vi "Paths to Commands_new.vi"(2 "Path":T4(array[cluster]), 3 "Path Properties":T1(array[cluster])=[{"Speed (um/s)"=0.4, "Direction"=0, "Orientation (For Filled)"=enum."Vertical", "Curve smooth Segments"=30.0, "Fill in spacing (um)"=0.3, "Start and End voltage"=[{"Numeric"=10.0, "Numeric 2"=10.0}, {"Numeric"=-10.0, "Numeric 2"=-10.0}, {"Numeric"=10.0, "Numeric 2"=10.0}], "Same Voltage"=TRUE, "Function Genrator?"=TRUE}, {"Speed (um/s)"=0.4, "Direction"=0, "Orientation (For Filled)"=enum."Vertical", "Curve smooth Segments"=30.0, "Fill in spacing (um)"=0.3, "Start and End voltage"=[{"Numeric"=10.0, "Numeric 2"=10.0}, {"Numeric"=-10.0, "Numeric 2"=-10.0}, {"Numeric"=10.0, "Numeric 2"=10.0}], "Same Voltage"=TRUE, "Function Genrator?"=TRUE}, {"Speed (um/s)"=0.4, "Direction"=0, "Orientation (For Filled)"=enum."Vertical", "Curve smooth Segments"=30.0, "Fill in spacing (um)"=0.3, "Start and End voltage"=[{"Numeric"=10.0, "Numeric 2"=10.0}, {"Numeric"=-10.0, "Numeric 2"=-10.0}, {"Numeric"=10.0, "Numeric 2"=10.0}], "Same Voltage"=TRUE, "Function Genrator?"=TRUE}, {"Speed (um/s)"=0.4, "Direction"=0, "Orientation (For Filled)"=enum."Vertical", "Curve smooth Segments"=30.0, "Fill in spacing (um)"=0.3, "Start and End voltage"=[{"Numeric"=10.0, "Numeric 2"=10.0}, {"Numeric"=-10.0, "Numeric 2"=-10.0}, {"Numeric"=10.0, "Numeric 2"=10.0}], "Same Voltage"=TRUE, "Function Genrator?"=TRUE}, {"Speed (um/s)"=0.4, "Direction"=0, "Orientation (For Filled)"=enum."Vertical", "Curve smooth Segments"=30.0, "Fill in spacing (um)"=0.3, "Start and End voltage"=[{"Numeric"=10.0, "Numeric 2"=10.0}, {"Numeric"=-10.0, "Numeric 2"=-10.0}, {"Numeric"=10.0, "Numeric 2"=10.0}], "Same Voltage"=TRUE, "Function Genrator?"=TRUE}, {"Speed (um/s)"=0.4, "Direction"=0, "Orientation (For Filled)"=enum."Vertical", "Curve smooth Segments"=30.0, "Fill in spacing (um)"=0.3, "Start and End voltage"=[{"Numeric"=10.0, "Numeric 2"=10.0}, {"Numeric"=-10.0, "Numeric 2"=-10.0}, {"Numeric"=10.0, "Numeric 2"=10.0}], "Same Voltage"=TRUE, "Function Genrator?"=TRUE}, {"Speed (um/s)"=0.4, "Direction"=0, "Orientation (For Filled)"=enum."Vertical", "Curve smooth Segments"=30.0, "Fill in spacing (um)"=0.3, "Start and End voltage"=[{"Numeric"=10.0, "Numeric 2"=10.0}, {"Numeric"=-10.0, "Numeric 2"=-10.0}, {"Numeric"=10.0, "Numeric 2"=10.0}], "Same Voltage"=TRUE, "Function Genrator?"=TRUE}, {"Speed (um/s)"=0.4, "Direction"=0, "Orientation (For Filled)"=enum."Vertical", "Curve smooth Segments"=30.0, "Fill in spacing (um)"=0.3, "Start and End voltage"=[{"Numeric"=10.0, "Numeric 2"=10.0}, {"Numeric"=-10.0, "Numeric 2"=-10.0}, {"Numeric"=10.0, "Numeric 2"=10.0}], "Same Voltage"=TRUE, "Function Genrator?"=TRUE}, {"Speed (um/s)"=0.4, "Direction"=0, "Orientation (For Filled)"=enum."Vertical", "Curve smooth Segments"=30.0, "Fill in spacing (um)"=0.3, "Start and End voltage"=[{"Numeric"=10.0, "Numeric 2"=10.0}, {"Numeric"=-10.0, "Numeric 2"=-10.0}, {"Numeric"=10.0, "Numeric 2"=10.0}], "Same Voltage"=TRUE, "Function Genrator?"=TRUE}, {"Speed (um/s)"=0.4, "Direction"=0, "Orientation (For Filled)"=enum."Vertical", "Curve smooth Segments"=30.0, "Fill in spacing (um)"=0.3, "Start and End voltage"=[{"Numeric"=10.0, "Numeric 2"=10.0}, {"Numeric"=-10.0, "Numeric 2"=-10.0}, {"Numeric"=10.0, "Numeric 2"=10.0}], "Same Voltage"=TRUE, "Function Genrator?"=TRUE}, {"Speed (um/s)"=0.4, "Direction"=0, "Orientation (For Filled)"=enum."Vertical", "Curve smooth Segments"=30.0, "Fill in spacing (um)"=0.3, "Start and End voltage"=[{"Numeric"=10.0, "Numeric 2"=10.0}, {"Numeric"=-10.0, "Numeric 2"=-10.0}, {"Numeric"=10.0, "Numeric 2"=10.0}], "Same Voltage"=TRUE, "Function Genrator?"=TRUE}, {"Speed (um/s)"=0.4, "Direction"=0, "Orientation (For Filled)"=enum."Vertical", "Curve smooth Segments"=30.0, "Fill in spacing (um)"=0.3, "Start and End voltage"=[{"Numeric"=10.0, "Numeric 2"=10.0}, {"Numeric"=-10.0, "Numeric 2"=-10.0}, {"Numeric"=10.0, "Numeric 2"=10.0}], "Same Voltage"=TRUE, "Function Genrator?"=TRUE}, {"Speed (um/s)"=0.4, "Direction"=0, "Orientation (For Filled)"=enum."Vertical", "Curve smooth Segments"=30.0, "Fill in spacing (um)"=0.3, "Start and End voltage"=[{"Numeric"=10.0, "Numeric 2"=10.0}, {"Numeric"=-10.0, "Numeric 2"=-10.0}, {"Numeric"=10.0, "Numeric 2"=10.0}], "Same Voltage"=TRUE, "Function Genrator?"=TRUE}, {"Speed (um/s)"=0.4, "Direction"=0, "Orientation (For Filled)"=enum."Vertical", "Curve smooth Segments"=30.0, "Fill in spacing (um)"=0.3, "Start and End voltage"=[{"Numeric"=10.0, "Numeric 2"=10.0}, {"Numeric"=-10.0, "Numeric 2"=-10.0}, {"Numeric"=10.0, "Numeric 2"=10.0}], "Same Voltage"=TRUE, "Function Genrator?"=TRUE}, {"Speed (um/s)"=0.4, "Direction"=0, "Orientation (For Filled)"=enum."Vertical", "Curve smooth Segments"=30.0, "Fill in spacing (um)"=0.3, "Start and End voltage"=[{"Numeric"=10.0, "Numeric 2"=10.0}, {"Numeric"=-10.0, "Numeric 2"=-10.0}, {"Numeric"=10.0, "Numeric 2"=10.0}], "Same Voltage"=TRUE, "Function Genrator?"=TRUE}, {"Speed (um/s)"=0.4, "Direction"=0, "Orientation (For Filled)"=enum."Vertical", "Curve smooth Segments"=30.0, "Fill in spacing (um)"=0.3, "Start and End voltage"=[{"Numeric"=10.0, "Numeric 2"=10.0}, {"Numeric"=-10.0, "Numeric 2"=-10.0}, {"Numeric"=10.0, "Numeric 2"=10.0}], "Same Voltage"=TRUE, "Function Genrator?"=TRUE}, {"Speed (um/s)"=0.4, "Direction"=0, "Orientation (For Filled)"=enum."Vertical", "Curve smooth Segments"=30.0, "Fill in spacing (um)"=0.3, "Start and End voltage"=[{"Numeric"=10.0, "Numeric 2"=10.0}, {"Numeric"=-10.0, "Numeric 2"=-10.0}, {"Numeric"=10.0, "Numeric 2"=10.0}], "Same Voltage"=TRUE, "Function Genrator?"=TRUE}, {"Speed (um/s)"=0.4, "Direction"=0, "Orientation (For Filled)"=enum."Vertical", "Curve smooth Segments"=30.0, "Fill in spacing (um)"=0.3, "Start and End voltage"=[{"Numeric"=10.0, "Numeric 2"=10.0}, {"Numeric"=-10.0, "Numeric 2"=-10.0}, {"Numeric"=10.0, "Numeric 2"=10.0}], "Same Voltage"=TRUE, "Function Genrator?"=TRUE}, {"Speed (um/s)"=0.4, "Direction"=0, "Orientation (For Filled)"=enum."Vertical", "Curve smooth Segments"=30.0, "Fill in spacing (um)"=0.3, "Start and End voltage"=[{"Numeric"=10.0, "Numeric 2"=10.0}, {"Numeric"=-10.0, "Numeric 2"=-10.0}, {"Numeric"=10.0, "Numeric 2"=10.0}], "Same Voltage"=TRUE, "Function Genrator?"=TRUE}, {"Speed (um/s)"=0.4, "Direction"=0, "Orientation (For Filled)"=enum."Vertical", "Curve smooth Segments"=30.0, "Fill in spacing (um)"=0.3, "Start and End voltage"=[{"Numeric"=10.0, "Numeric 2"=10.0}, {"Numeric"=-10.0, "Numeric 2"=-10.0}, {"Numeric"=10.0, "Numeric 2"=10.0}], "Same Voltage"=TRUE, "Function Genrator?"=TRUE}, {"Speed (um/s)"=0.4, "Direction"=0, "Orientation (For Filled)"=enum."Vertical", "Curve smooth Segments"=30.0, "Fill in spacing (um)"=0.3, "Start and End voltage"=[{"Numeric"=10.0, "Numeric 2"=10.0}, {"Numeric"=-10.0, "Numeric 2"=-10.0}, {"Numeric"=10.0, "Numeric 2"=10.0}], "Same Voltage"=TRUE, "Function Genrator?"=TRUE}, {"Speed (um/s)"=0.4, "Direction"=0, "Orientation (For Filled)"=enum."Vertical", "Curve smooth Segments"=30.0, "Fill in spacing (um)"=0.3, "Start and End voltage"=[{"Numeric"=10.0, "Numeric 2"=10.0}, {"Numeric"=-10.0, "Numeric 2"=-10.0}, {"Numeric"=10.0, "Numeric 2"=10.0}], "Same Voltage"=TRUE, "Function Genrator?"=TRUE}, {"Speed (um/s)"=0.4, "Direction"=0, "Orientation (For Filled)"=enum."Vertical", "Curve smooth Segments"=30.0, "Fill in spacing (um)"=0.3, "Start and End voltage"=[{"Numeric"=10.0, "Numeric 2"=10.0}, {"Numeric"=-10.0, "Numeric 2"=-10.0}, {"Numeric"=10.0, "Numeric 2"=10.0}], "Same Voltage"=TRUE, "Function Genrator?"=TRUE}, {"Speed (um/s)"=0.4, "Direction"=0, "Orientation (For Filled)"=enum."Vertical", "Curve smooth Segments"=30.0, "Fill in spacing (um)"=0.3, "Start and End voltage"=[{"Numeric"=10.0, "Numeric 2"=10.0}, {"Numeric"=-10.0, "Numeric 2"=-10.0}, {"Numeric"=10.0, "Numeric 2"=10.0}], "Same Voltage"=TRUE, "Function Genrator?"=TRUE}, {"Speed (um/s)"=0.4, "Direction"=0, "Orientation (For Filled)"=enum."Vertical", "Curve smooth Segments"=30.0, "Fill in spacing (um)"=0.3, "Start and End voltage"=[{"Numeric"=10.0, "Numeric 2"=10.0}, {"Numeric"=-10.0, "Numeric 2"=-10.0}, {"Numeric"=10.0, "Numeric 2"=10.0}], "Same Voltage"=TRUE, "Function Genrator?"=TRUE}, {"Speed (um/s)"=0.4, "Direction"=0, "Orientation (For Filled)"=enum."Vertical", "Curve smooth Segments"=30.0, "Fill in spacing (um)"=0.3, "Start and End voltage"=[{"Numeric"=10.0, "Numeric 2"=10.0}, {"Numeric"=-10.0, "Numeric 2"=-10.0}, {"Numeric"=10.0, "Numeric 2"=10.0}], "Same Voltage"=TRUE, "Function Genrator?"=TRUE}, {"Speed (um/s)"=0.4, "Direction"=0, "Orientation (For Filled)"=enum."Vertical", "Curve smooth Segments"=30.0, "Fill in spacing (um)"=0.3, "Start and End voltage"=[{"Numeric"=10.0, "Numeric 2"=10.0}, {"Numeric"=-10.0, "Numeric 2"=-10.0}, {"Numeric"=10.0, "Numeric 2"=10.0}], "Same Voltage"=TRUE, "Function Genrator?"=TRUE}, {"Speed (um/s)"=0.4, "Direction"=0, "Orientation (For Filled)"=enum."Vertical", "Curve smooth Segments"=30.0, "Fill in spacing (um)"=0.3, "Start and End voltage"=[{"Numeric"=10.0, "Numeric 2"=10.0}, {"Numeric"=-10.0, "Numeric 2"=-10.0}, {"Numeric"=10.0, "Numeric 2"=10.0}], "Same Voltage"=TRUE, "Function Genrator?"=TRUE}, {"Speed (um/s)"=0.4, "Direction"=0, "Orientation (For Filled)"=enum."Vertical", "Curve smooth Segments"=30.0, "Fill in spacing (um)"=0.3, "Start and End voltage"=[{"Numeric"=10.0, "Numeric 2"=10.0}, {"Numeric"=-10.0, "Numeric 2"=-10.0}, {"Numeric"=10.0, "Numeric 2"=10.0}], "Same Voltage"=TRUE, "Function Genrator?"=TRUE}, {"Speed (um/s)"=0.4, "Direction"=0, "Orientation (For Filled)"=enum."Vertical", "Curve smooth Segments"=30.0, "Fill in spacing (um)"=0.3, "Start and End voltage"=[{"Numeric"=10.0, "Numeric 2"=10.0}, {"Numeric"=-10.0, "Numeric 2"=-10.0}, {"Numeric"=10.0, "Numeric 2"=10.0}], "Same Voltage"=TRUE, "Function Genrator?"=TRUE}] {"Direction" items=["Forward", "Backward"]}, 4 "error in (no error)":errorcluster) -> (0 "Lithography information":T2(array[cluster]), 1 "error out":errorcluster)   [LabVIEW 2013]
doc: "This VI processes the rectangles' data and outputs lithography data."
uses:
  <vilib>/Analysis/Matrix/Datatypes/RealMatrix.ctl
  Global Variables.vi
  <vilib>/Analysis/Matrix/NI_Matrix.lvlib
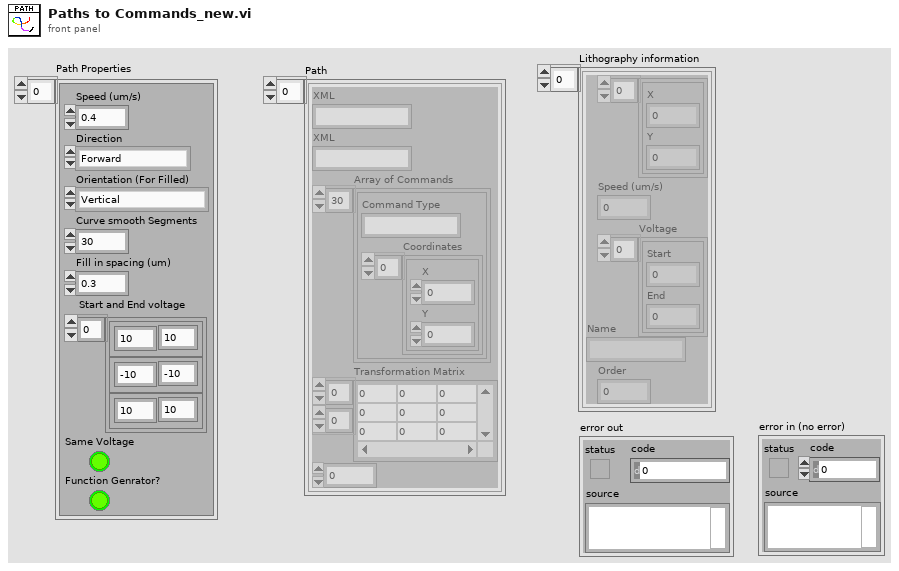
[diagram p1: front panel]
types:
  T1 = cluster{"Speed (um/s)":dbl, "Direction":u16, "Orientation (For Filled)":enum16{"Horizontal", "Vertical"}, "Curve smooth Segments":dbl, "Fill in spacing (um)":dbl, "Start and End voltage":cluster{"Numeric":dbl, "Numeric 2":dbl}[], "Same Voltage":bool, "Function Genrator?":bool}[]
  T2 = cluster{cluster{"X":dbl, "Y":dbl}[], "Speed (um/s)":dbl, "Voltage":cluster{"Start":dbl, "End":dbl}[], "Name":string, "Order":i32}[]
  T3 = typedef "NI_Matrix.lvlib/RealMatrix.ctl" = dbl[][]
  T4 = cluster{"XML":string, "XML":string, "Array of Commands":cluster{"Command Type":string, "Coordinates":cluster{"X":dbl, "Y":dbl}[]}[], "Transformation Matrix":T3, "Order":i32}[]
  T5 = cluster{"Command Type":string, "Coordinates":cluster{"X":dbl, "Y":dbl}[]}[]
  T6 = cluster{"Command Type":string, "Coordinates":cluster{"X":dbl, "Y":dbl}[]}
  T7 = cluster{"Horizontal X":dbl, "Horizontal X":dbl}[]
  T8 = cluster{cluster{"X":dbl, "Y":dbl}[], "Speed (um/s)":dbl, "Voltage":cluster{"Numeric":dbl, "Numeric 2":dbl}[], string, "Order":i32}
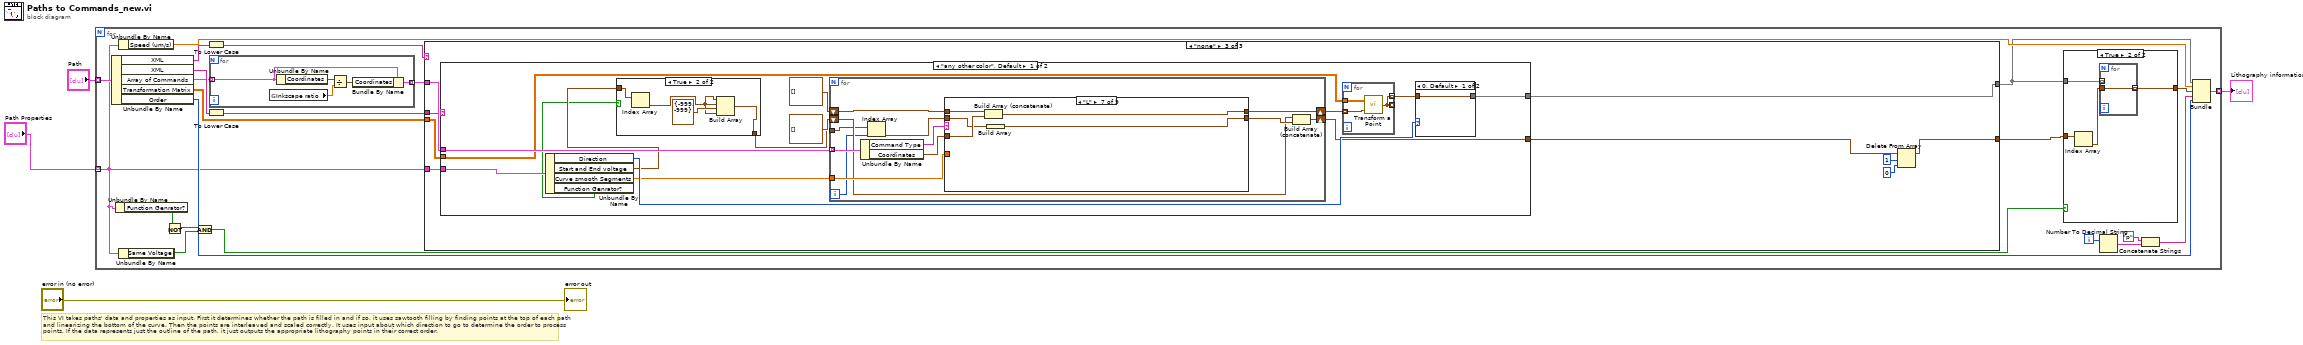
[diagram p0: block diagram]
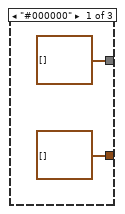
[diagram p3: hidden frame]
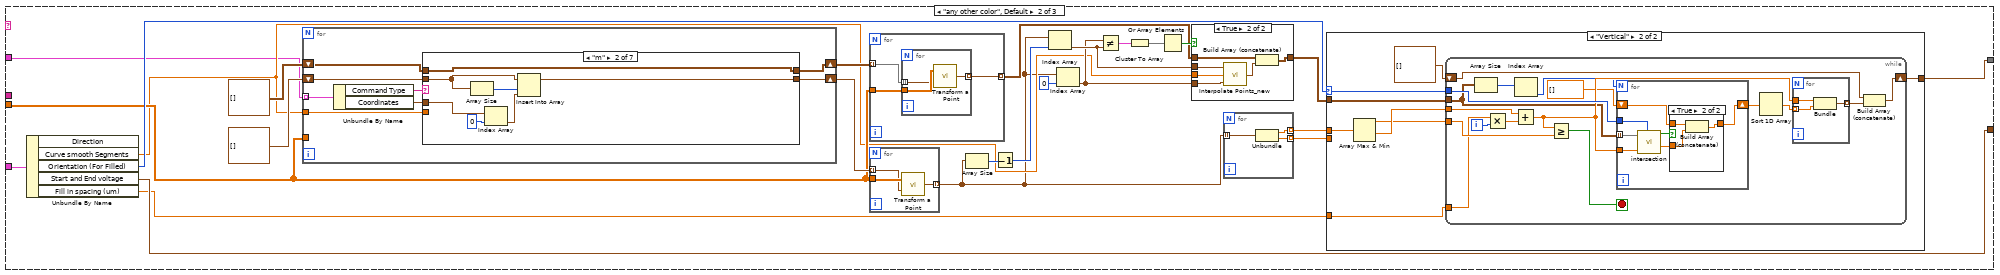
[diagram p4: hidden frame]
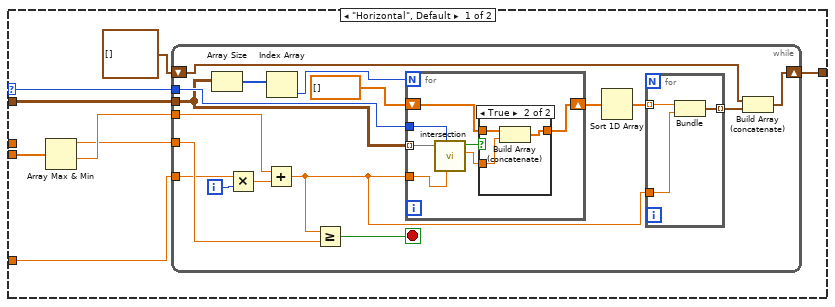
[diagram p5: hidden frame]
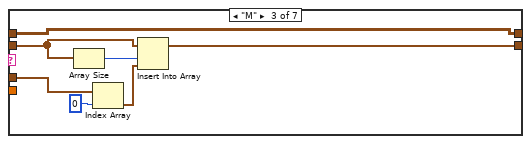
[diagram p10: hidden frame]
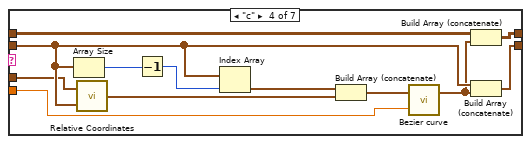
[diagram p11: hidden frame]
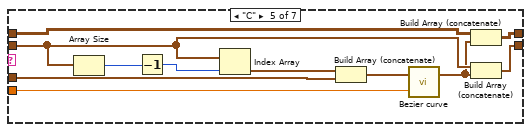
[diagram p12: hidden frame]
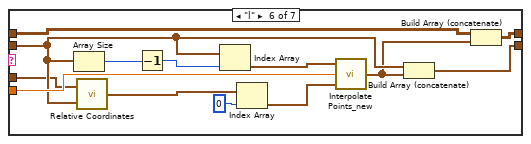
[diagram p13: hidden frame]
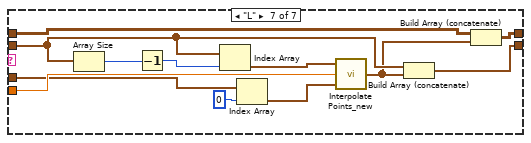
[diagram p14: hidden frame]
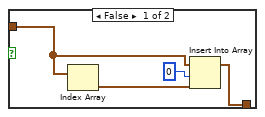
[diagram p15: hidden frame]
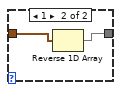
[diagram p16: hidden frame]
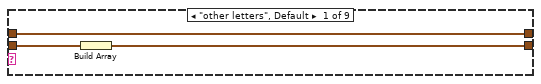
[diagram p17: hidden frame]
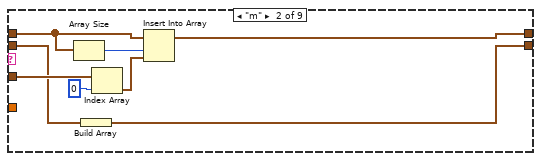
[diagram p18: hidden frame]
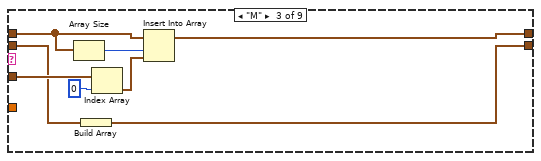
[diagram p19: hidden frame]
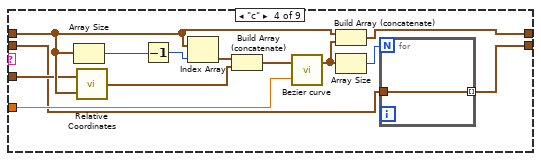
[diagram p20: hidden frame]
diagram:
  # "This VI takes paths' data and properties as input. First it determines whether the path is filled in and if so, it uses sawtooth filling by finding points at the top of each path \nand linearizing the bottom of the curve. Then the points are interleaved and scaled correctly. It uses input about which direction to go to determine the order to process \npoints. If the data represents just the outline of the path, it just outputs the appropriate lithography points in their correct order."
  n1 = for {
    tunnel: "Path" -> [w22] mode=indexing
    tunnel: "Path Properties" -> [w9] mode=indexing
    tunnel: [w13] -> w2 mode=indexing
    i -> [w18]
    n2 = Unbundle By Name(w22) -> ("XML"=w27:string, "XML"=w25:string, "Array of Commands"=w15:T5, "Transformation Matrix"=w17:T3, "Order"=w16:i32)
    n3 = Unbundle By Name(w9) -> ("Function Genrator?"=w8:bool)
    n4 = Unbundle By Name(w9) -> ("Speed (um/s)"=w23:dbl)
    n5 = Unbundle By Name(w9) -> ("Same Voltage"=w6:bool)
    n6 = Not(x=w8) -> (.not. x?=w7:bool)
    n7 = And(x=w7, y=w6) -> (x .and. y?=w5:bool)
    n8 = To Lower Case(string=w27) -> (all lower case string=w26:string)
    n9 = To Lower Case(string=w25) -> (all lower case string=w24:string)
    n10 = for {
      tunnel: w15 -> [w35] mode=indexing
      tunnel: [w34] -> w14 mode=indexing
      n11 = global read "Global Variables.vi" "Inkscape ratio"() -> (w37:dbl)
      n12 = Unbundle By Name(w35) -> ("Coordinates"=w38:cluster{"X":dbl, "Y":dbl}[])
      n13 = Divide(x=w38, y=w37) -> (x/y=w36:cluster{"X":dbl, "Y":dbl}[])
      n14 = Bundle By Name(cluster=w35, "Coordinates"=w36) -> (w34:T6)
    }
    n15 = case shown="\"none\"" w26 {
      tunnel: w24 -> [_ _ w239]
      tunnel: w9 -> [_ w64 w242]
      tunnel: [cluster{"X":dbl, "Y":dbl}[] [] w51 w241] -> w12
      tunnel: w14 -> [_ w41 w243]
      tunnel: w17 -> [_ w47 w240]
      tunnel: [cluster{"Numeric":dbl, "Numeric 2":dbl}[] [] ("Voltage") w63 w235] -> w10
      frame "#000000" {
      }
      frame "any other color", Default {
        n16 = Unbundle By Name(w64) -> ("Curve smooth Segments"=w44:dbl, "Orientation (For Filled)"=w54:enum16{"Horizontal", "Vertical"}, "Start and End voltage"=w63:cluster{"Numeric":dbl, "Numeric 2":dbl}[], "Fill in spacing (um)"=w42:dbl)  [unwired: 1 out]
        n17 = for {
          tunnel: w41 -> [w163] mode=indexing
          shift-right: [w167] -> w62
          shift-left: cluster{"X":dbl, "Y":dbl}[] [] -> [w169]
          tunnel: w44 -> [w168]
          tunnel: w47 -> [_]
          shift-right: [w165] -> w46
          shift-left: cluster{"X":dbl, "Y":dbl}[][] [] -> [w164]
          n18 = Unbundle By Name(w163) -> ("Command Type"=w170:string, "Coordinates"=w166:cluster{"X":dbl, "Y":dbl}[])
          n19 = case shown="\"m\"" w170 {
            tunnel: w166 -> [_ w174 w181 w190 w204 w213 w226]
            tunnel: w169 -> [w172 w176 w182 w198 w209 w215 w227]
            tunnel: [w172 w177 w183 w192 w205 w221 w233] -> w167
            tunnel: w168 -> [_ _ _ w191 w200 w222 w234]
            tunnel: [w171 w173 w180 w189 w202 w211 w225] -> w165
            tunnel: w164 -> [w171 w173 w180 w187 w201 w210 w223]
            frame "other letters", Default {
            }
            frame "m" {
              n20 = Array Size(array=w176) -> (size(s)=w179:i32)
              n21 = Index Array(array=w174, index=0) -> (element=w178:cluster{"X":dbl, "Y":dbl})
              n22 = Insert Into Array(array=w176, index=w179, new element=w178) -> (w177:cluster{"X":dbl, "Y":dbl}[])
            }
            frame "M" {
              n23 = Array Size(array=w182) -> (size(s)=w185:i32)
              n24 = Index Array(array=w181, index=0) -> (element=w184:cluster{"X":dbl, "Y":dbl})
              n25 = Insert Into Array(array=w182, index=w185, new element=w184) -> (w183:cluster{"X":dbl, "Y":dbl}[])
            }
            frame "c" {
              n26 = Array Size(array=w198) -> (size(s)=w194:i32)
              n27 = call "Relative Coordinates.vi"("All Coordinates"=w198, "Command Coordinates"=w190) -> ("Adjusted Command Coordinates"=w196:cluster{"X":dbl, "Y":dbl}[])
              n28 = Decrement(x=w194) -> (x-1=w193:i32)
              n29 = Index Array(array=w198, index=w193) -> (element=w197:cluster{"X":dbl, "Y":dbl})
              n30 = Build Array (concatenate)(w197, w196) -> (w195:cluster{"X":dbl, "Y":dbl}[])
              n31 = call "Bezier curve.vi"("Segments"=w191, "Parameters"=w195) -> ("Coordinate Array"=w188:cluster{"X":dbl, "Y":dbl}[])  [unwired: 1 out]
              n32 = Build Array (concatenate)(w187, w188) -> (w189:cluster{"X":dbl, "Y":dbl}[][])
              n33 = Build Array (concatenate)(w198, w188) -> (w192:cluster{"X":dbl, "Y":dbl}[])
            }
            frame "C" {
              n34 = Array Size(array=w209) -> (size(s)=w207:i32)
              n35 = Decrement(x=w207) -> (x-1=w206:i32)
              n36 = Index Array(array=w209, index=w206) -> (element=w208:cluster{"X":dbl, "Y":dbl})
              n37 = Build Array (concatenate)(w208, w204) -> (w199:cluster{"X":dbl, "Y":dbl}[])
              n38 = call "Bezier curve.vi"("Segments"=w200, "Parameters"=w199) -> ("Coordinate Array"=w203:cluster{"X":dbl, "Y":dbl}[])  [unwired: 1 out]
              n39 = Build Array (concatenate)(w201, w203) -> (w202:cluster{"X":dbl, "Y":dbl}[][])
              n40 = Build Array (concatenate)(w209, w203) -> (w205:cluster{"X":dbl, "Y":dbl}[])
            }
            frame "l" {
              n41 = Array Size(array=w215) -> (size(s)=w217:i32)
              n42 = call "Relative Coordinates.vi"("All Coordinates"=w215, "Command Coordinates"=w213) -> ("Adjusted Command Coordinates"=w220:cluster{"X":dbl, "Y":dbl}[])
              n43 = Decrement(x=w217) -> (x-1=w216:i32)
              n44 = Index Array(array=w215, index=w216) -> (element=w219:cluster{"X":dbl, "Y":dbl})
              n45 = Index Array(array=w220, index=0) -> (element=w218:cluster{"X":dbl, "Y":dbl})
              n46 = call "Interpolate Points_new.vi"("End Point"=w218, "Points number"=w222, "Start Point"=w219) -> ("Output Point Array"=w212:cluster{"X":dbl, "Y":dbl}[])
              n47 = Build Array (concatenate)(w215, w212) -> (w221:cluster{"X":dbl, "Y":dbl}[])
              n48 = Build Array (concatenate)(w210, w212) -> (w211:cluster{"X":dbl, "Y":dbl}[][])
            }
            frame "L" {
              n49 = Array Size(array=w227) -> (size(s)=w229:i32)
              n50 = Decrement(x=w229) -> (x-1=w228:i32)
              n51 = Index Array(array=w227, index=w228) -> (element=w232:cluster{"X":dbl, "Y":dbl})
              n52 = Index Array(array=w226, index=0) -> (element=w230:cluster{"X":dbl, "Y":dbl})
              n53 = call "Interpolate Points_new.vi"("End Point"=w230, "Points number"=w234, "Start Point"=w232) -> ("Output Point Array"=w224:cluster{"X":dbl, "Y":dbl}[])
              n54 = Build Array (concatenate)(w227, w224) -> (w233:cluster{"X":dbl, "Y":dbl}[])
              n55 = Build Array (concatenate)(w223, w224) -> (w225:cluster{"X":dbl, "Y":dbl}[][])
            }
          }
        }
        n56 = for {
          tunnel: [w66] -> w45 mode=indexing
          tunnel: w47 -> [w68]
          tunnel: w46 -> [w67] mode=indexing
          n57 = for {
            tunnel: w68 -> [w71]
            tunnel: w67 -> [w70] mode=indexing
            tunnel: [w69] -> w66 mode=indexing
            n58 = call "Transform a Point.vi"("Point to Transform"=w70, "Transformation Matrix"=w71) -> ("Transformed Point"=w69:cluster{"X":dbl, "Y":dbl})
          }
        }
        n59 = for {
          tunnel: [w160] -> w43 mode=indexing
          tunnel: w47 -> [w162]
          tunnel: w62 -> [w161] mode=indexing
          n60 = call "Transform a Point.vi"("Point to Transform"=w161, "Transformation Matrix"=w162) -> ("Transformed Point"=w160:cluster{"X":dbl, "Y":dbl})
        }
        n61 = Array Size(array=w43) -> (size(s)=w59:i32)
        n62 = Decrement(x=w59) -> (x-1=w50:i32)
        n63 = Index Array(array=w43, index=w50) -> (element=w56:cluster{"X":dbl, "Y":dbl})
        n64 = Index Array(array=w43, index=0) -> (element=w55:cluster{"X":dbl, "Y":dbl})
        n65 = Not Equal?(x=w55, y=w56) -> (x != y?=w58:cluster{"X":bool, "Y":bool})
        n66 = Cluster To Array(cluster=w58) -> (array=w57:bool[])
        n67 = Or Array Elements(Boolean array=w57) -> (logical OR=w48:bool)
        n68 = case shown="True" w48 {
          tunnel: w45 -> [w153 w156]
          tunnel: w56 -> [_ w158]
          tunnel: w55 -> [_ w157]
          tunnel: [w153 w159] -> w52
          tunnel: w44 -> [_ w154]
          frame False {
          }
          frame True {
            n69 = call "Interpolate Points_new.vi"("End Point"=w157, "Points number"=w154, "Start Point"=w158) -> ("Output Point Array"=w155:cluster{"X":dbl, "Y":dbl}[])
            n70 = Build Array (concatenate)(w156, w155) -> (w159:cluster{"X":dbl, "Y":dbl}[][])
          }
        }
        n71 = for {
          tunnel: w43 -> [w74] mode=indexing
          tunnel: [w73] -> w49 mode=indexing
          tunnel: [w72] -> w53 mode=indexing
          n72 = Unbundle(w74) -> ("X"=w73:dbl, "Y"=w72:dbl)
        }
        n73 = case shown="\"Vertical\"" w54 {
          selector: w54 -> [w78 w116]
          tunnel: w53 -> [w82 _]
          tunnel: w52 -> [w79 w117]
          tunnel: [w77 w118] -> w51
          tunnel: w49 -> [_ w115]
          tunnel: w42 -> [w75 w114]
          frame "Horizontal", Default {
            n74 = Array Max & Min(array=w82) -> (max value=w80:dbl, min value=w81:dbl)  [unwired: 2 out]
            n75 = while {
              tunnel: w81 -> [w99]
              tunnel: w80 -> [w96]
              tunnel: w79 -> [w87]
              tunnel: w78 -> [w94]
              shift-right: [w89] -> w77
              shift-left: cluster{"Horizontal X":dbl, dbl}[] [] -> [w88]
              tunnel: w75 -> [w83]
              i -> [w98]
              stop <- w95 stop-if-true
              n76 = Array Size(array=w87) -> (size(s)=w86:i32[])
              n77 = Multiply(x=w83, y=w98) -> (x*y=w97:dbl)
              n78 = Add(x=w99, y=w97) -> (x+y=w91:dbl)
              n79 = Index Array(array=w86) -> (element=w85:i32)  [unwired: 1 in]
              n80 = Greater Or Equal?(x=w91, y=w96) -> (x >= y?=w95:bool)
              n81 = for {
                N: w85 -> [_]
                tunnel: w87 -> [w109] mode=indexing
                tunnel: w94 -> [w108]
                tunnel: w91 -> [w107]
                shift-right: [w104] -> w93
                shift-left: dbl[] [] -> [w103]
                n82 = call "intersection.vi"("Coordinate Array"=w109, "Enum"=w108, "Horizontal Y"=w107) -> ("intersection"=w106:bool, "Horizontal X"=w105:dbl)  [unwired: 2 in, 2 out]
                n83 = case shown="True" w106 {
                  tunnel: w105 -> [_ w113]
                  tunnel: [w110 w112] -> w104
                  tunnel: w103 -> [w110 w111]
                  frame False {
                  }
                  frame True {
                    n84 = Build Array (concatenate)(w111, w113) -> (w112:dbl[])
                  }
                }
              }
              n85 = Sort 1D Array(array=w93) -> (sorted array=w92:dbl[])
              n86 = for {
                tunnel: w92 -> [w102] mode=indexing
                tunnel: w91 -> [w101]
                tunnel: [w100] -> w90 mode=indexing
                n87 = Bundle("Horizontal X"=w102, w101) -> (w100:cluster{"Horizontal X":dbl, dbl})  [unwired: 1 in]
              }
              n88 = Build Array (concatenate)(w88, w90) -> (w89:cluster{"Horizontal X":dbl, dbl}[])
            }
          }
          frame "Vertical" {
            n89 = Array Max & Min(array=w115) -> (max value=w120:dbl, min value=w121:dbl)  [unwired: 2 out]
            n90 = while {
              tunnel: w121 -> [w138]
              tunnel: w120 -> [w135]
              tunnel: w117 -> [w126]
              tunnel: w116 -> [w133]
              shift-right: [w128] -> w118
              shift-left: cluster{"Horizontal X":dbl, dbl}[] [] -> [w127]
              tunnel: w114 -> [w122]
              i -> [w137]
              stop <- w134 stop-if-true
              n91 = Array Size(array=w126) -> (size(s)=w125:i32[])
              n92 = Multiply(x=w122, y=w137) -> (x*y=w136:dbl)
              n93 = Add(x=w138, y=w136) -> (x+y=w130:dbl)
              n94 = Index Array(array=w125) -> (element=w124:i32)  [unwired: 1 in]
              n95 = Greater Or Equal?(x=w130, y=w135) -> (x >= y?=w134:bool)
              n96 = for {
                N: w124 -> [_]
                tunnel: w126 -> [w148] mode=indexing
                tunnel: w133 -> [w147]
                tunnel: w130 -> [w143]
                shift-right: [w145] -> w132
                shift-left: dbl[] [] -> [w144]
                n97 = call "intersection.vi"("Coordinate Array"=w148, "Enum"=w147, "Vertical X"=w143) -> ("intersection"=w146:bool, "Vertical Y"=w142:dbl)  [unwired: 2 in, 2 out]
                n98 = case shown="True" w146 {
                  tunnel: w142 -> [_ w152]
                  tunnel: [w149 w151] -> w145
                  tunnel: w144 -> [w149 w150]
                  frame False {
                  }
                  frame True {
                    n99 = Build Array (concatenate)(w150, w152) -> (w151:dbl[])
                  }
                }
              }
              n100 = Sort 1D Array(array=w132) -> (sorted array=w131:dbl[])
              n101 = for {
                tunnel: w131 -> [w140] mode=indexing
                tunnel: w130 -> [w139]
                tunnel: [w141] -> w129 mode=indexing
                n102 = Bundle(w139, "Horizontal X"=w140) -> (w141:cluster{dbl, "Horizontal X":dbl})  [unwired: 1 in]
              }
              n103 = Build Array (concatenate)(w127, w129) -> (w128:T7)
            }
          }
        }
      }
      frame "none" {
        n104 = case shown="\"any other color\", Default" w239 {
          tunnel: w243 -> [w257 _]
          tunnel: w242 -> [w255 _]
          tunnel: [w254 cluster{"X":dbl, "Y":dbl}[] []] -> w241
          tunnel: w240 -> [w251 _]
          tunnel: [w248 cluster{"Numeric":dbl, "Numeric 2":dbl}[] [] ("Voltage")] -> w236
          frame "any other color", Default {
            n105 = Unbundle By Name(w255) -> ("Direction"=w253:u16, "Start and End voltage"=w245:cluster{"Numeric":dbl, "Numeric 2":dbl}[], "Curve smooth Segments"=w252:dbl, "Function Genrator?"=w244:bool)
            n106 = case shown="True" w244 {
              tunnel: [w259 w263] -> w246
              tunnel: w245 -> [w258 w265]
              frame False {
                n107 = Index Array(array=w258) -> (element=w260:cluster{"Numeric":dbl, "Numeric 2":dbl})  [unwired: 1 in]
                n108 = Insert Into Array(array=w258, index=0, new element=w260) -> (w259:cluster{"Numeric":dbl, "Numeric 2":dbl}[])
              }
              frame True {
                n109 = Index Array(array=w265) -> (element=w262:cluster{"Numeric":dbl, "Numeric 2":dbl})  [unwired: 1 in]
                n110 = Build Array(w262, w262, cluster{"Numeric":i32, "Numeric 2":i32} {"Numeric"=-999, "Numeric 2"=-999} ("Voltage"), w262) -> (w263:cluster{"Numeric":dbl, "Numeric 2":dbl}[])
              }
            }
            n111 = for {
              tunnel: w257 -> [w283] mode=indexing
              shift-right: [w279] -> w250
              shift-left: cluster{"X":dbl, "Y":dbl}[] [] -> [w280]
              tunnel: w252 -> [w278]
              tunnel: w246 -> [w274]
              shift-right: [w276] -> w248
              shift-left: cluster{"Numeric":dbl, "Numeric 2":dbl}[] [] -> [w275]
              i -> [w273]
              n112 = Unbundle By Name(w283) -> ("Command Type"=w282:string, "Coordinates"=w281:cluster{"X":dbl, "Y":dbl}[])
              n113 = Index Array(array=w274, index=w273) -> (element=w272:cluster{"Numeric":dbl, "Numeric 2":dbl})
              n114 = case shown="\"L\"" w282 {
                tunnel: w281 -> [_ w289 w297 w307 w321 w332 w338 _ _]
                tunnel: w280 -> [w286 w290 w298 w314 w327 w334 w340 w343 w350]
                tunnel: [w286 w291 w299 w315 w328 w333 w339 w344 w351] -> w279
                tunnel: w278 -> [_ _ _ w308 w322 _ _ _ _]
                tunnel: w272 -> [w285 w288 w296 w305 w319 w331 w337 w342 w349]
                tunnel: [w284 w287 w295 w303 w318 w330 w336 w341 w348] -> w277
                frame "other letters", Default {
                  n115 = Build Array(w285) -> (w284:cluster{"Numeric":dbl, "Numeric 2":dbl}[])
                }
                frame "m" {
                  n116 = Array Size(array=w290) -> (size(s)=w293:i32)
                  n117 = Build Array(w288) -> (w287:cluster{"Numeric":dbl, "Numeric 2":dbl}[])
                  n118 = Index Array(array=w289, index=0) -> (element=w292:cluster{"X":dbl, "Y":dbl})
                  n119 = Insert Into Array(array=w290, index=w293, new element=w292) -> (w291:cluster{"X":dbl, "Y":dbl}[])
                }
                frame "M" {
                  n120 = Array Size(array=w298) -> (size(s)=w301:i32)
                  n121 = Build Array(w296) -> (w295:cluster{"Numeric":dbl, "Numeric 2":dbl}[])
                  n122 = Index Array(array=w297, index=0) -> (element=w300:cluster{"X":dbl, "Y":dbl})
                  n123 = Insert Into Array(array=w298, index=w301, new element=w300) -> (w299:cluster{"X":dbl, "Y":dbl}[])
                }
                frame "c" {
                  n124 = Array Size(array=w314) -> (size(s)=w310:i32)
                  n125 = call "Relative Coordinates.vi"("All Coordinates"=w314, "Command Coordinates"=w307) -> ("Adjusted Command Coordinates"=w312:cluster{"X":dbl, "Y":dbl}[])
                  n126 = Decrement(x=w310) -> (x-1=w309:i32)
                  n127 = Index Array(array=w314, index=w309) -> (element=w313:cluster{"X":dbl, "Y":dbl})
                  n128 = Build Array (concatenate)(w313, w312) -> (w311:cluster{"X":dbl, "Y":dbl}[])
                  n129 = call "Bezier curve.vi"("Segments"=w308, "Parameters"=w311) -> ("Coordinate Array"=w306:cluster{"X":dbl, "Y":dbl}[])  [unwired: 1 out]
                  n130 = Build Array (concatenate)(w314, w306) -> (w315:cluster{"X":dbl, "Y":dbl}[])
                  n131 = Array Size(array=w306) -> (size(s)=w304:i32)
                  n132 = for {
                    N: w304 -> [_]
                    tunnel: w305 -> [w316]
                    tunnel: [w316] -> w303 mode=indexing
                  }
                }
                frame "C" {
                  n133 = Array Size(array=w327) -> (size(s)=w324:i32)
                  n134 = Decrement(x=w324) -> (x-1=w323:i32)
                  n135 = Index Array(array=w327, index=w323) -> (element=w326:cluster{"X":dbl, "Y":dbl})
                  n136 = Build Array (concatenate)(w326, w321) -> (w325:cluster{"X":dbl, "Y":dbl}[])
                  n137 = call "Bezier curve.vi"("Segments"=w322, "Parameters"=w325) -> ("Coordinate Array"=w320:cluster{"X":dbl, "Y":dbl}[])  [unwired: 1 out]
                  n138 = Build Array (concatenate)(w327, w320) -> (w328:cluster{"X":dbl, "Y":dbl}[])
                  n139 = Array Size(array=w320) -> (size(s)=w317:i32)
                  n140 = for {
                    N: w317 -> [_]
                    tunnel: w319 -> [w329]
                    tunnel: [w329] -> w318 mode=indexing
                  }
                }
                frame "l" {
                  n141 = call "Relative Coordinates.vi"("All Coordinates"=w334, "Command Coordinates"=w332) -> ("Adjusted Command Coordinates"=w335:cluster{"X":dbl, "Y":dbl}[])
                  n142 = Build Array(w331) -> (w330:cluster{"Numeric":dbl, "Numeric 2":dbl}[])
                  n143 = Build Array (concatenate)(w334, w335) -> (w333:cluster{"X":dbl, "Y":dbl}[])
                }
                frame "L" {
                  n144 = Build Array (concatenate)(w340, w338) -> (w339:cluster{"X":dbl, "Y":dbl}[])
                  n145 = Build Array(w337) -> (w336:cluster{"Numeric":dbl, "Numeric 2":dbl}[])
                }
                frame "z" {
                  n146 = Array Size(array=w343) -> (size(s)=w346:i32)
                  n147 = Build Array(w342) -> (w341:cluster{"Numeric":dbl, "Numeric 2":dbl}[])
                  n148 = Index Array(array=w343, index=0) -> (element=w345:cluster{"X":dbl, "Y":dbl})
                  n149 = Insert Into Array(array=w343, index=w346, new element=w345) -> (w344:cluster{"X":dbl, "Y":dbl}[])
                }
                frame "Z" {
                  n150 = Array Size(array=w350) -> (size(s)=w353:i32)
                  n151 = Build Array(w349) -> (w348:cluster{"Numeric":dbl, "Numeric 2":dbl}[])
                  n152 = Index Array(array=w350, index=0) -> (element=w352:cluster{"X":dbl, "Y":dbl})
                  n153 = Insert Into Array(array=w350, index=w353, new element=w352) -> (w351:cluster{"X":dbl, "Y":dbl}[])
                }
              }
              n154 = Build Array (concatenate)(w275, w277) -> (w276:cluster{"Numeric":dbl, "Numeric 2":dbl}[])
            }
            n155 = for {
              tunnel: [w266] -> _ mode=indexing
              tunnel: w251 -> [w268]
              tunnel: w250 -> [w267] mode=indexing
              tunnel: [w266] -> w249 mode=indexing
              n156 = call "Transform a Point.vi"("Point to Transform"=w267, "Transformation Matrix"=w268) -> ("Transformed Point"=w266:cluster{"X":dbl, "Y":dbl})
            }
            n157 = case shown="0, Default" w253 {
              tunnel: [w269 w270] -> w254
              tunnel: w249 -> [w269 w271]
              frame 0, Default {
              }
              frame 1 {
                n158 = Reverse 1D Array(array=w271) -> (reversed array=w270:cluster{"X":dbl, "Y":dbl}[])
              }
            }
          }
          frame "#000000" {
          }
        }
        n159 = Delete From Array(array=w236, length=1, index=0) -> (array with subset deleted=w235:cluster{"Numeric":dbl, "Numeric 2":dbl}[])  [unwired: 1 out]
      }
    }
    n160 = case shown="True" w5 {
      tunnel: w12 -> [_ w32]
      tunnel: w10 -> [w28 w31]
      tunnel: [w28 w29] -> w11
      frame False {
      }
      frame True {
        n161 = Index Array(array=w31) -> (element=w30:cluster{"Numeric":dbl, "Numeric 2":dbl})  [unwired: 1 in]
        n162 = for {
          tunnel: w32 -> [_] mode=indexing
          tunnel: [w33] -> w29 mode=indexing
          tunnel: w30 -> [w33]
        }
      }
    }
    n163 = Number To Decimal String(number=w18) -> (decimal integer string=w20:string)  [unwired: 1 in]
    n164 = Concatenate Strings("p", w20) -> (w19:string)
    n165 = Bundle(w12, "Speed (um/s)"=w23, "Voltage"=w11, w19, "Order"=w16) -> (w13:T8)  [unwired: 1 in]
  }
  "Lithography information" <- w2
  "error out" <- "error in (no error)"
